vi "CountSetup.vi"(11 "real report 3":refnum<vi>) -> (2 "cont setup":i32, 3 "real report 4":refnum<vi>)   [LabVIEW 2018]
panel:
  in  "real report 2":i32(listbox) caption="real report"
  in  "error in (no error)":errorcluster caption="错误输入（无错误）"
  out "error out":errorcluster caption="错误输出"
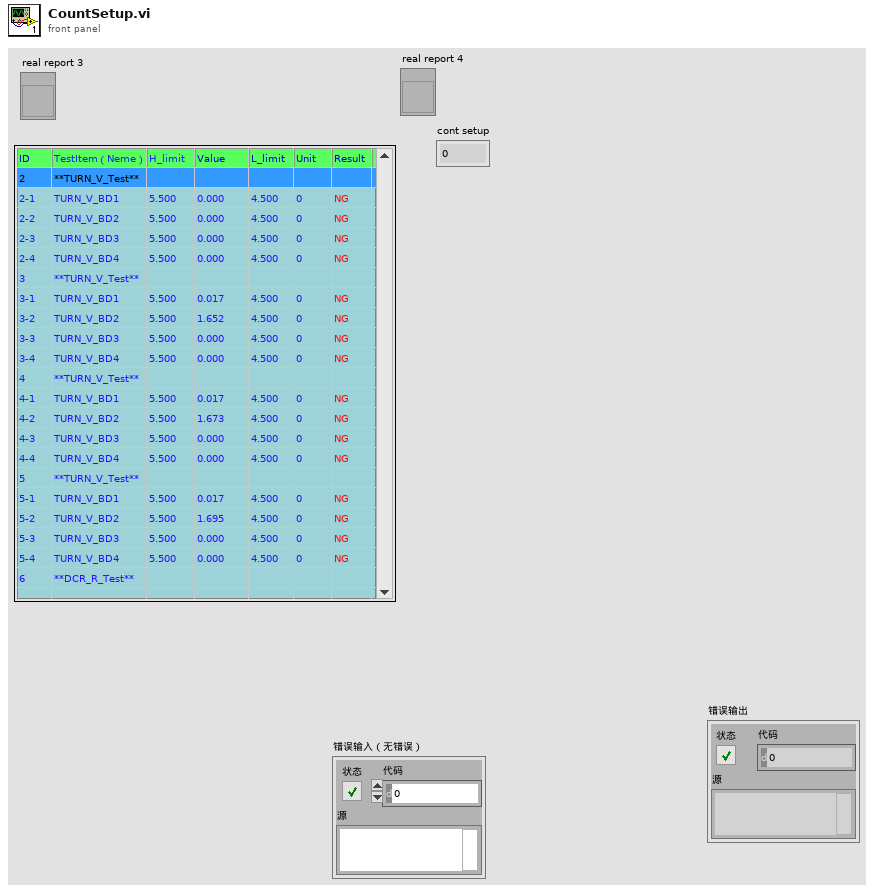
[diagram p1: front panel]
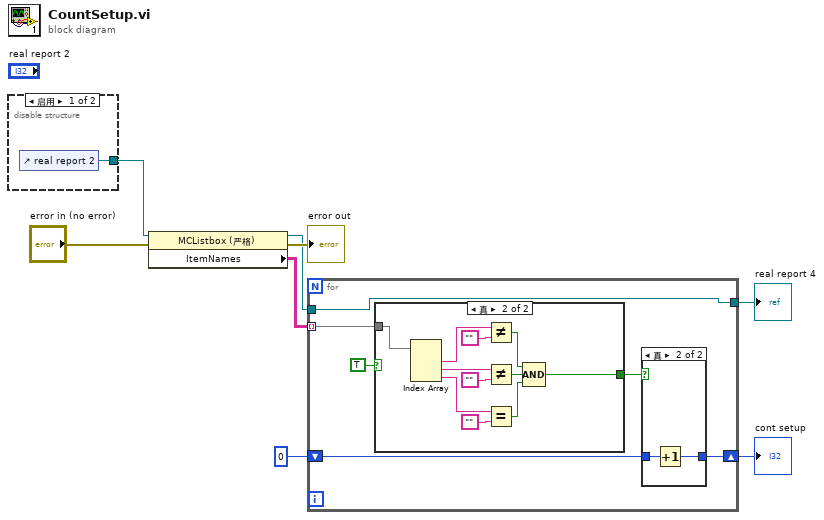
[diagram p0: block diagram]
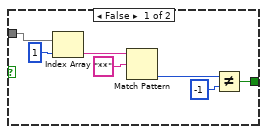
[diagram p2: hidden frame]
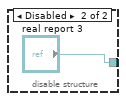
[diagram p4: hidden frame]
diagram:
  n1 = disable-structure shown="启用" {
    disable-tunnel: [w9 "real report 3"] -> w3
    frame Enabled {
      n2 = control-ref of="real report 2"() -> (w9:refnum<vi>)
    }
    frame Disabled {
    }
  }
  n3 = property class="MCListbox (严格)"(reference=w3, error in="error in (no error)") -> (reference out=w6:refnum<vi>, error out=→"error out":errorcluster, "ItemNames"=w4:string[][])
  n4 = for {
    tunnel: w4 -> [w12] mode=indexing
    shift-right: [w15] -> w2
    shift-left: 0 -> [w16]
    tunnel: [w14] -> w1
    tunnel: w6 -> [w14]
    n5 = case shown="真" TRUE {
      tunnel: w12 -> [w18 w34]
      tunnel: [w19 w28] -> w13
      frame False {
        n6 = Index Array(array=w18, index=1 ("索引")) -> (element=w17:string)
        n7 = Match Pattern(string=w17, regular expression="**" ("正则表达式")) -> (offset past match=w23:i32)  [unwired: 1 in, 3 out]
        n8 = Not Equal?(x=w23, y=-1) -> (x != y?=w19:bool)
      }
      frame True {
        n9 = Index Array(array=w34) -> (element #1=w33:string, element #2=w31:string, element #3=w25:string)  [unwired: 3 in]
        n10 = Not Equal?(x=w33, y="") -> (x != y?=w30:bool)
        n11 = Not Equal?(x=w31, y="") -> (x != y?=w29:bool)
        n12 = Equal?(x=w25, y="") -> (x = y?=w24:bool)
        n13 = Compound Arithmetic op=AND ("复合运算")(w30, w29, w24) -> (w28:bool)
      }
    }
    n14 = case shown="真" w13 {
      tunnel: w16 -> [w35 w37]
      tunnel: [w35 w36] -> w15
      frame False {
      }
      frame True {
        n15 = Increment(x=w37) -> (x+1=w36:i32)
      }
    }
  }
  "cont setup" <- w2
  "real report 4" <- w1
